vi "MultiplyMatrices.vi"(1 "Matrix2":string[][](array[string])=[["1", "0", "0", "0"], ["-1/f", "1", "0", "0"], ["0", "0", "1", "0"], ["0", "0", "-1/f", "1"]], 2 "Matrix1":string[][](array[string])=[["1", "0", "0", "0"], ["-1/f", "1", "0", "0"], ["0", "0", "1", "0"], ["0", "0", "-1/f", "1"]]) -> (0 "Matrix3":string[][](array[string])=[["1", "0", "0", "0"], ["-1/f", "1", "0", "0"], ["0", "0", "1", "0"], ["0", "0", "-1/f", "1"]])   [LabVIEW 2011]
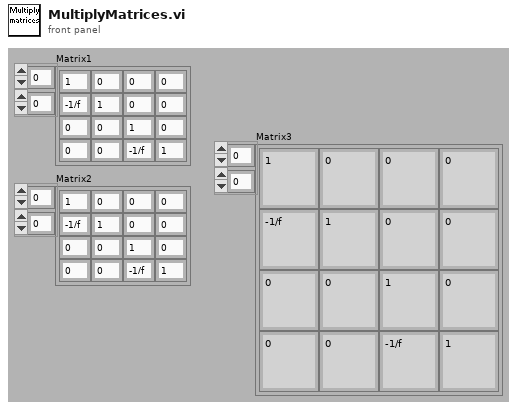
[diagram p1: front panel]
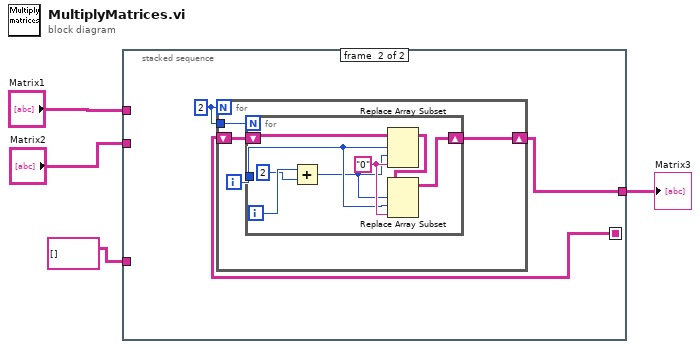
[diagram p0: block diagram]
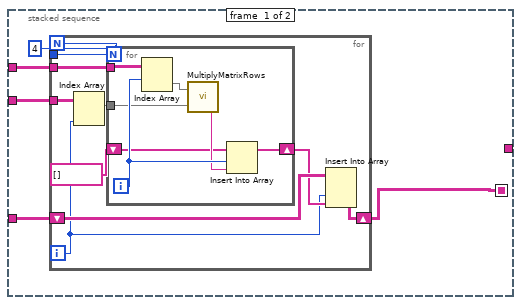
[diagram p2: hidden frame]
diagram:
  n1 = stacked-sequence {
    seq-local: [w5 _] -> [_ w27]
    tunnel: "Matrix1" -> [w8 _]
    tunnel: "Matrix2" -> [w7 _]
    tunnel: string[][] [] -> [w6 _]
    tunnel: [_ w26] -> w1
    frame #0 {
      w9 = 4
      n2 = for {
        N: w9 -> [_]
        tunnel: w9 -> [w18]
        tunnel: w8 -> [w17]
        tunnel: w7 -> [w14]
        shift-right: [w10] -> w5
        shift-left: w6 -> [w13]
        i -> [w11]
        n3 = Index Array(array=w14, index (col)=w11) -> (element=w15:string[])  [unwired: 1 in]
        n4 = for {
          N: w18 -> [_]
          tunnel: w17 -> [w25]
          shift-right: [w20] -> w12
          shift-left: string[] [] -> [w21]
          tunnel: w15 -> [w19]
          i -> [w23]
          n5 = Index Array(array=w25, index (row)=w23) -> (element=w24:string[])  [unwired: 1 in]
          n6 = call "MultiplyMatrixRows.vi"("Column"=w19, "Row"=w24) -> ("Output"=w22:string)
          n7 = Insert Into Array(array=w21, index=w23, new element=w22) -> (w20:string[])
        }
        n8 = Insert Into Array(array=w13, index (col)=w11, new element=w12) -> (w10:string[][])  [unwired: 1 in]
      }
    }
    frame #1 {
      w28 = 2
      n9 = for {
        N: w28 -> [_]
        shift-right: [w30] -> w26
        shift-left: w27 -> [w32]
        tunnel: w28 -> [w29]
        i -> [w31]
        n10 = for {
          N: w29 -> [_]
          tunnel: w31 -> [w34]
          shift-right: [w35] -> w30
          shift-left: w32 -> [w40]
          i -> [w39]
          w36 = "0" ("new element/subarray")
          n11 = Add(x=w39, y=2) -> (x+y=w33:i32)
          n12 = Replace Array Subset(array=w40, new element=w36, index (row)=w34, index (col)=w33) -> (w37:string[][])
          n13 = Replace Array Subset(array=w37, new element=w36, index (row)=w33, index (col)=w34) -> (w35:string[][])
        }
      }
    }
  }
  "Matrix3" <- w1
